vi "Error Handler.vi"(8 "error in (no error)":errorcluster) -> (0 "error out":errorcluster)   [LabVIEW 2011, in "Sliding Menu Library.lvlib"]
uses:
  Sliding Menu Library.lvlib
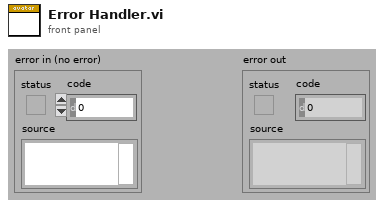
[diagram p1: front panel]
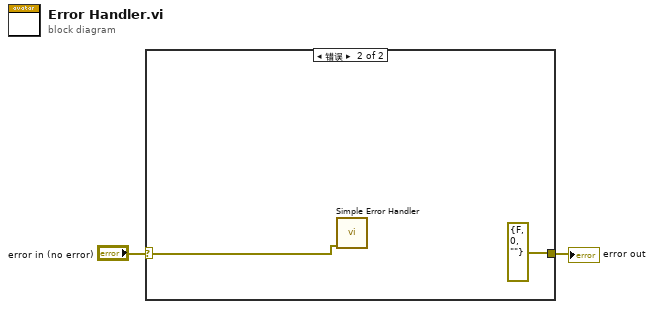
[diagram p0: block diagram]
diagram:
  n1 = case shown="错误" "error in (no error)" {
    selector: "error in (no error)" -> [w3 w4]
    tunnel: [w3 errorcluster {"status"=FALSE, "code"=0, "source"=""} ("error IO")] -> w2
    frame No Error {
    }
    frame Error {
      n2 = call <vilib>:"Simple Error Handler.vi"("error in (no error)"=w4) -> ()  [unwired: 4 in, 5 out]
    }
  }
  "error out" <- w2
